vi "Write_ProcessConfig_State.vi"(8 "error in (no error)":errorcluster, 10 "State":T1(ring)=enum."Closed", 11 "Process in":refnum<class "Process.lvclass">) -> (0 "error out":errorcluster, 3 "Process out":refnum<class "Process.lvclass">)   [LabVIEW 2013, in "Process.lvclass"]
uses:
  Process.lvclass
  Process.lvclass/Process.ctl
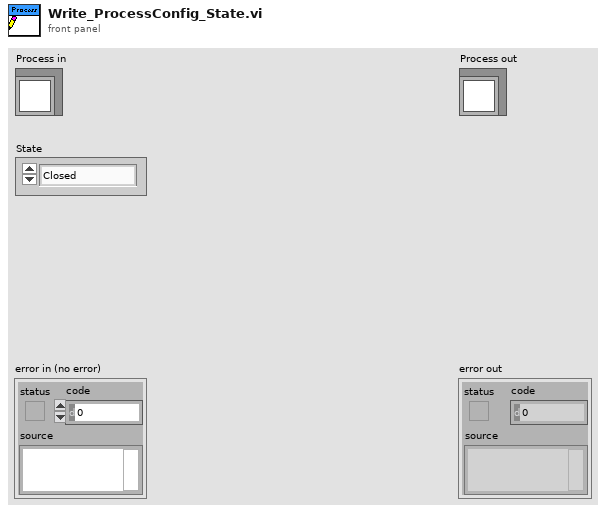
[diagram p1: front panel]
types:
  T1 = enum32{"Invalid", "Standard", "Closed", "Hidden", "Minimized", "Maximized"}
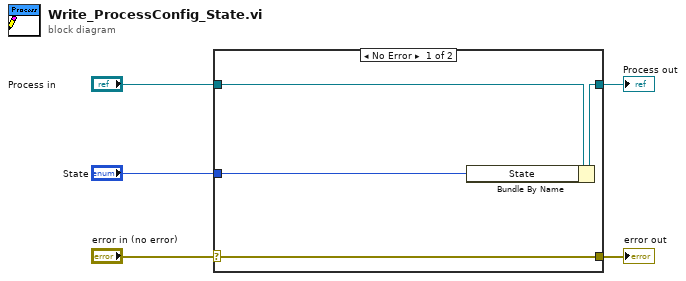
[diagram p0: block diagram]
diagram:
  n1 = case shown="No Error" "error in (no error)" {
    selector: "error in (no error)" -> [w9 w10]
    tunnel: [w9 w10] -> w4
    tunnel: [w7 w11] -> w2
    tunnel: "Process in" -> [w8 w11]
    tunnel: "State" -> [w6 _]
    frame No Error {
      n2 = Bundle By Name(cluster=w8, "State"=w6) -> (w7:refnum<class "Process.lvclass">)
    }
    frame Error {
    }
  }
  "error out" <- w4
  "Process out" <- w2
